vi "AngleFurtherFromRobot.vi"(10 "Angle 2":dbl, 11 "Angle 1":T1) -> (3 "Angle further from Robot":T1)   [LabVIEW 2011]
doc: "Exactly as the title says. It takes in two angles and finds the angle that's closer to the robot's current heading."
uses:
  2 Typedefs/apparent wind direction.ctl
  2 Globals/2 Global.vi
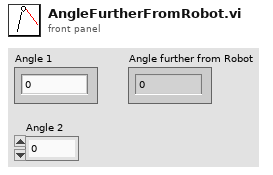
[diagram p1: front panel]
types:
  T1 = typedef "apparent wind direction.ctl" = dbl
  T2 = typedef "heading.ctl" = dbl
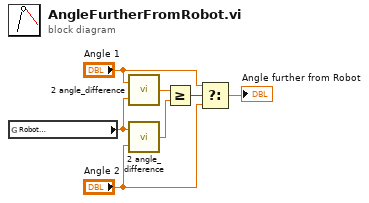
[diagram p0: block diagram]
diagram:
  n1 = global read "2 Global.vi" "Robot\nHeading"() -> (w3:T2)
  n2 = call "2 angle_difference.vi"("Angle 2"=w3, "Angle 1"="Angle 1") -> ("Difference"=w2:dbl)
  n3 = call "2 angle_difference.vi"("Angle 2"="Angle 2", "Angle 1"=w3) -> ("Difference"=w4:dbl)
  n4 = Greater Or Equal?(x=w2, y=w4) -> (x >= y?=w1:bool)
  n5 = Select(t="Angle 1", s=w1, f="Angle 2") -> (s? t:f=→"Angle further from Robot":T1)
